vi "Read from Machine.vi"(8 "error in (no error)":errorcluster, 11 "Machine In":refnum<visa-resource-name>) -> (0 "error out":errorcluster, 2 "read buffer":string, 3 "Machine Out":refnum<visa-resource-name>)   [LabVIEW 2017]
doc: "Reads machine response from USB connection.\n\n<B>Inputs</B>: \n- Machine In: Specifies the desired machine connected to computer via USB.\n- Error In: Reads error (if any) from previous vi. \n\n<B>Outputs</B>: \n- Machine Out: Reference to the selected USB device.\n- Read Buffer: Returns the machine's response (string). \n- Error Out: Returns an error if one occurs in vi (or has occurred in a previous vi), and passes it to next wired terminal."
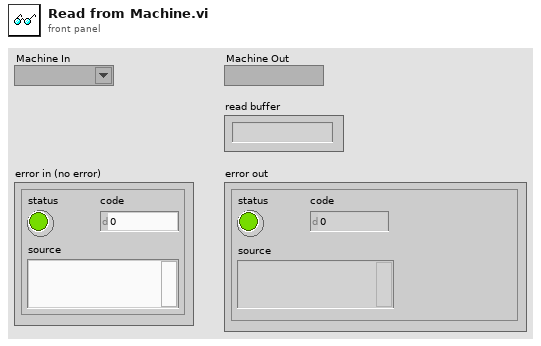
[diagram p1: front panel]
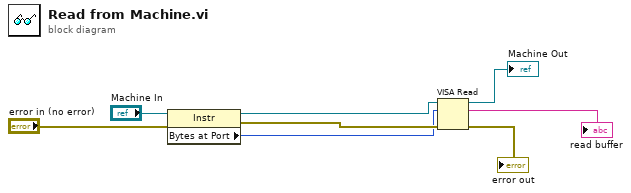
[diagram p0: block diagram]
diagram:
  n1 = property class="Instr"(reference="Machine In", error in="error in (no error)") -> (reference out=w2:refnum<visa-resource-name>, error out=w3:errorcluster, "Bytes at Port"=w1:u32)
  n2 = VISA Read(VISA resource name=w2, byte count=w1, error in (no error)=w3) -> (VISA resource name out=→"Machine Out":refnum<visa-resource-name>, read buffer=→"read buffer":string, error out=→"error out":errorcluster)  [unwired: 1 out]
